vi "Set Group Property.vi"(5 "Value":variant, 7 "Name":string, 8 "error in (no error)":errorcluster, 10 "Group Name":string, 11 "TDMS Log File Specification in":refnum<class "TDMS Log File Specification.lvclass">) -> (0 "error out":errorcluster, 3 "TDMS Log File Specification out":refnum<class "TDMS Log File Specification.lvclass">)   [LabVIEW 2015, in "Waveform Data Logger Shared.lvlib" / "TDMS Log File Specification.lvclass"]
uses:
  TDMS Log File Specification.lvclass
  TDMS Log File Specification.lvclass/TDMS Log File Specification.ctl
  Property Specification.ctl
  Channel Group Specification.ctl
  Channel Specification.ctl
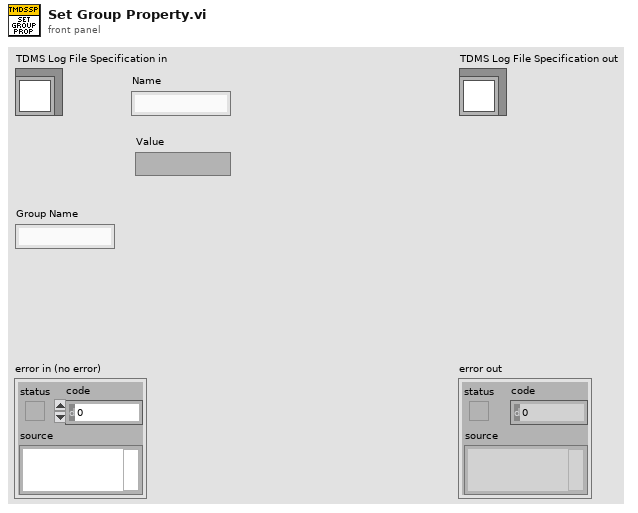
[diagram p1: front panel]
types:
  T1 = typedef "Waveform Data Logger Shared.lvlib/TDMS Log File Specification.lvclass/Property Specification.ctl" = cluster{"Name":string, "Value":variant}
  T2 = typedef "Waveform Data Logger Shared.lvlib/TDMS Log File Specification.lvclass/Channel Group Specification.ctl" = cluster{"Name":string, "Properties":T1[], "Channels":T3[]}
  T3 = typedef "Waveform Data Logger Shared.lvlib/TDMS Log File Specification.lvclass/Channel Specification.ctl" = cluster{"Name":string, "Properties":T1[]}
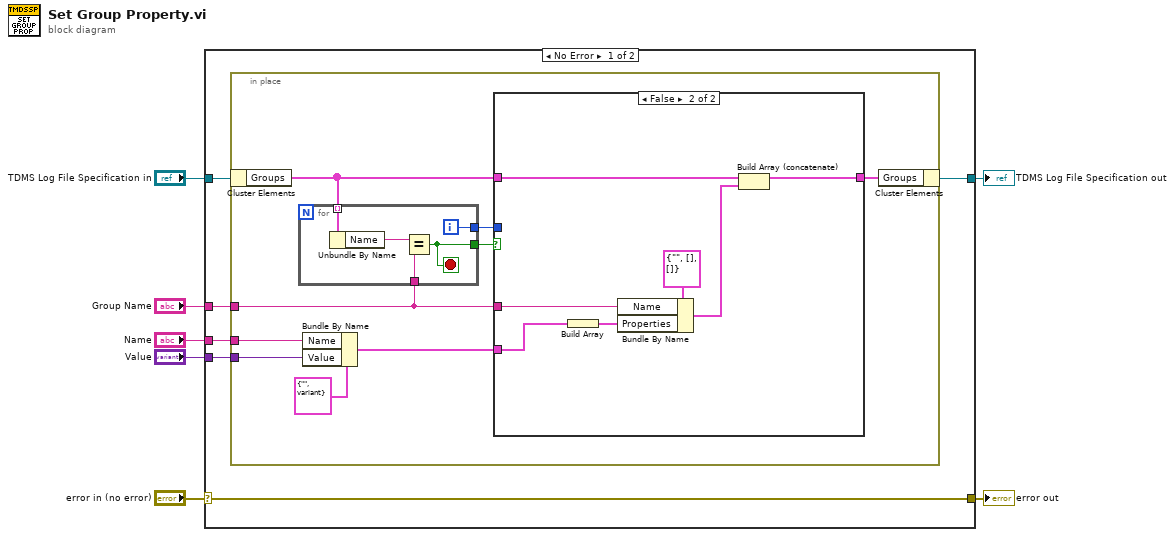
[diagram p0: block diagram]
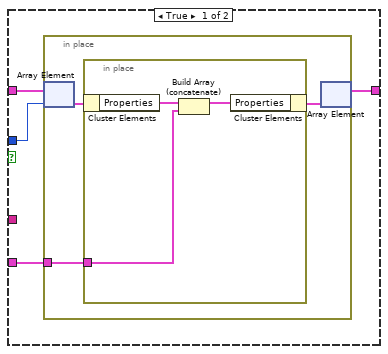
[diagram p2: hidden frame]
diagram:
  n1 = case shown="No Error" "error in (no error)" {
    selector: "error in (no error)" -> [w13 w46]
    tunnel: [w13 w46] -> w6
    tunnel: [w9 w45] -> w4
    tunnel: "TDMS Log File Specification in" -> [w12 w45]
    tunnel: "Name" -> [w11 _]
    tunnel: "Value" -> [w10 _]
    tunnel: "Group Name" -> [w8 _]
    frame No Error {
      n2 = in-place {
        in-place-border: w11 -> [w21]
        in-place-border: w10 -> [w20]
        in-place-border: w8 -> [w14]
        n3 = in-place-cluster #1(w12) -> ("Groups"=w17:T2[])
        n4 = for {
          tunnel: w17 -> [w44] mode=indexing
          tunnel: w14 -> [w42]
          tunnel: [w41] -> w19
          tunnel: [w40] -> w18
          i -> [w40]
          stop <- w41 stop-if-true
          n5 = Unbundle By Name(w44) -> ("Name"=w43:string)
          n6 = Equal?(x=w43, y=w42) -> (x = y?=w41:bool)
        }
        n7 = Bundle By Name(cluster=T1 {"Name"="", "Value"=variant} ("Property"), "Name"=w21, "Value"=w20) -> (w16:T1)
        n8 = case shown="False" w19 {
          tunnel: w18 -> [w25 _]
          tunnel: w17 -> [w26 w38]
          tunnel: w16 -> [w24 w39]
          tunnel: [w23 w37] -> w15
          tunnel: w14 -> [_ w34]
          frame True {
            n9 = in-place {
              in-place-border: w24 -> [w28]
              n10 = in-place-array #2(w26, w25) -> (w29:T2)
              n11 = in-place {
                in-place-border: w28 -> [w30]
                n12 = in-place-cluster #3(w29) -> ("Properties"=w32:T1[])
                n13 = Build Array (concatenate)(w32, w30) -> (w31:T1[])
                n14 = in-place-cluster #3("Properties"=w31) -> (w27:T2)
              }
              n15 = in-place-array #2(w27) -> (w23:T2[])  [unwired: 1 out]
            }
          }
          frame False {
            n16 = Build Array(w39) -> (w36:T1[])
            n17 = Bundle By Name(cluster=T2 {"Name"="", "Properties"=[], "Channels"=[]} ("Group Specification"), "Name"=w34, "Properties"=w36) -> (w33:T2)
            n18 = Build Array (concatenate)(w38, w33) -> (w37:T2[])
          }
        }
        n19 = in-place-cluster #1("Groups"=w15) -> (w9:refnum<class "TDMS Log File Specification.lvclass">)
      }
    }
    frame Error {
    }
  }
  "error out" <- w6
  "TDMS Log File Specification out" <- w4
